vi "constructor.vi"(8 "error in (no error)":errorcluster, 11 "builder settings":T1) -> (0 "error out":errorcluster, 3 "Builders":refnum<class "Builder.lvclass">)   [LabVIEW 2024, in "Builder.lvclass"]
uses:
  Builder.lvclass
  Builder.lvclass/Builder.ctl
  <vilib>/regexp/Match Regular Expression.xnode
  packed_library/PackedLibrary.lvclass
  builder settings.ctl
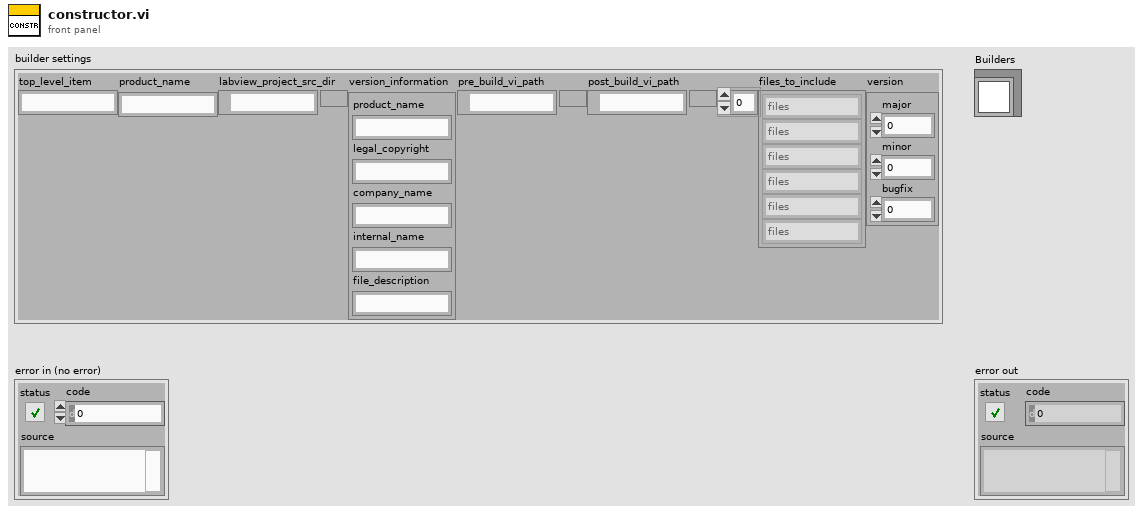
[diagram p1: front panel]
types:
  T1 = typedef "Builder.lvclass/builder settings.ctl" = cluster{"top_level_item":string, "product_name":string, "labview_project_src_dir":path, "version_information":cluster{"product_name":string, "legal_copyright":string, "company_name":string, "internal_name":string, "file_description":string}, "pre_build_vi_path":path, "post_build_vi_path":path, "files_to_include":string[], "version":cluster{"major":u16, "minor":u16, "bugfix":u16}}
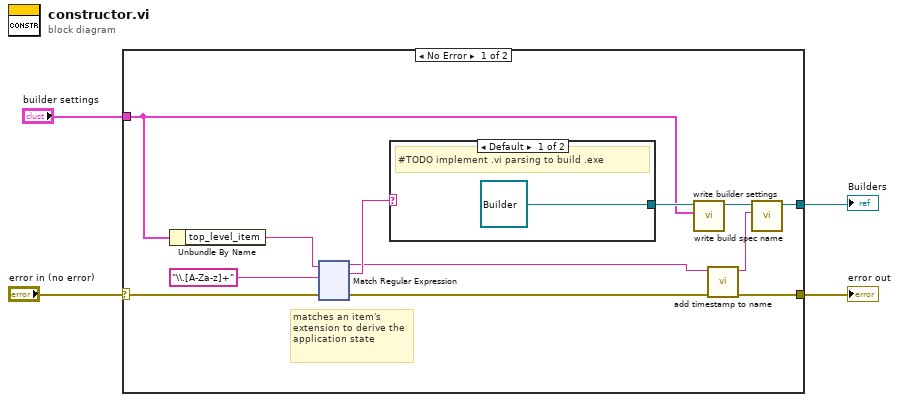
[diagram p0: block diagram]
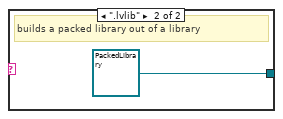
[diagram p2: hidden frame]
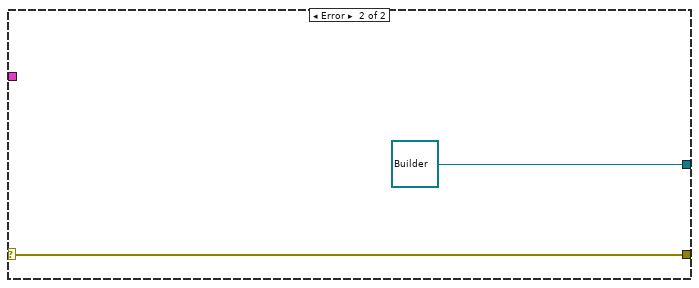
[diagram p3: hidden frame]
diagram:
  n1 = case shown="No Error" "error in (no error)" {
    selector: "error in (no error)" -> [w13 w137]
    tunnel: [w16 w137] -> w4
    tunnel: [w5 refnum<class "Builder.lvclass"> refnum ("Builders out")] -> w2
    tunnel: "builder settings" -> [w6 _]
    frame No Error {
      # "matches an item's extension to derive the application state"
      n2 = Unbundle By Name(w6) -> ("top_level_item"=w7:string)
      n3 = xnode "Match Regular Expression"("input string"=w7, "regular expression"="\\.[A-Za-z]+", "error in"=w13) -> ("before match"=w9:string, "whole match"=w15:string, "error out"=w12:errorcluster)  [unwired: 3 in, 2 out]
      n4 = case shown="Default" w15 {
        tunnel: [refnum<class "Builder.lvclass"> refnum ("Builders") refnum<class "PackedLibrary.lvclass"> refnum ("PackedLibrary.lvclass")] -> w14
        frame Default {
          # "#TODO implement .vi parsing to build .exe"
        }
        frame ".lvlib" {
          # "builds a packed library out of a library"
        }
      }
      n5 = call "write builder settings.vi"("builder settings"=w6, "Builder in"=w14) -> ("Builder out"=w10:refnum<class "Builder.lvclass">)  [unwired: 9 in]
      n6 = call "add timestamp to name.vi"("error in (no error)"=w12, "name"=w9) -> ("error out"=w16:errorcluster, "build spec name"=w11:string)  [unwired: 8 in]
      n7 = call "write build spec name.vi"("build spec name"=w11, "Builders in"=w10) -> ("Builders out"=w5:refnum<class "Builder.lvclass">)  [unwired: 9 in]
    }
    frame Error {
    }
  }
  "error out" <- w4
  "Builders" <- w2
